vi "pop_nil.vi"(8 "error in (no error)":errorcluster, 11 "Lua in":refnum<class "Lua.lvclass">) -> (0 "error out":errorcluster, 2 "value (ignored)":bool, 3 "Lua out":refnum<class "Lua.lvclass">)   [LabVIEW 2020, in "Lua for LabVIEW.lvlib" / "Lua.lvclass"]
doc: "Pop any value from the stack without returning the result."
uses:
  Lua.lvclass
  Lua.lvclass/Lua.ctl
  lib/lua.dll/lua.dll.lvlib
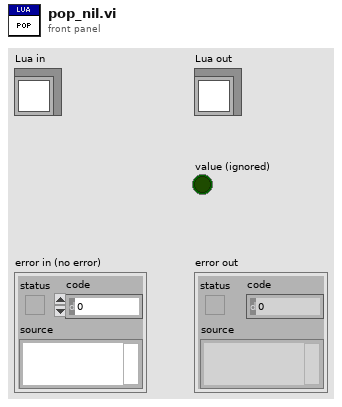
[diagram p1: front panel]
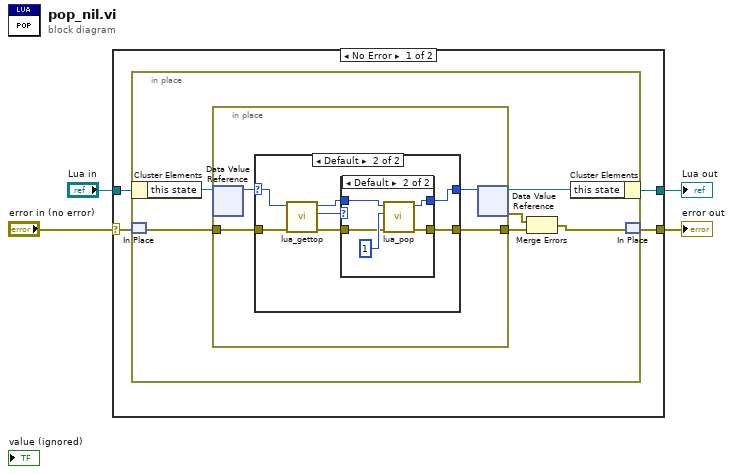
[diagram p0: block diagram]
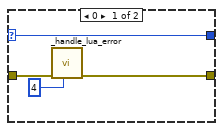
[diagram p2: hidden frame]
diagram:
  n1 = case shown="No Error" "error in (no error)" {
    selector: "error in (no error)" -> [w5 w38]
    tunnel: [w6 w38] -> w3
    tunnel: [w7 w37] -> w1
    tunnel: "Lua in" -> [w8 w37]
    frame No Error {
      n2 = in-place {
        n3 = in-place-cluster #1(w8) -> ("this state"=w13:refnum<data-value>)
        n4 = in-place-match #2(w5) -> (w14:errorcluster)
        n5 = in-place {
          in-place-border: w14 -> [w18]
          in-place-border: [w15] -> w9
          n6 = in-place-dvr #3(w13) -> (w17:u64)  [unwired: 1 out]
          n7 = case shown="Default" w17 {
            selector: w17 -> [w22 w26]
            tunnel: [w22 w28] -> w16
            tunnel: w18 -> [w19 w27]
            tunnel: [w20 w29] -> w15
            frame 0 {
              n8 = call "_handle_lua_error.vi"("lua status"=4 ("lua_load errcode"), "error in (no error)"=w19) -> ("error out"=w20:errorcluster)  [unwired: 9 in]
            }
            frame Default {
              n9 = call "lua_gettop.vi"("error in (no error)"=w27, "lua_state_p"=w26) -> ("error out"=w25:errorcluster, "index"=w24:i32, "lua_state_p out"=w23:u64)  [unwired: 7 in]
              n10 = case shown="Default" w24 {
                tunnel: [w31 w36] -> w29
                tunnel: [w30 w35] -> w28
                tunnel: w25 -> [w31 w33]
                tunnel: w23 -> [w30 w32]
                frame 0 {
                }
                frame Default {
                  n11 = call "lua_pop.vi"("error in (no error)"=w33, "n"=1 ("index"), "lua_state_p"=w32) -> ("error out"=w36:errorcluster, "lua_state_p out"=w35:u64)  [unwired: 7 in]
                }
              }
            }
          }
          n12 = in-place-dvr #3(w16) -> (w12:refnum<data-value>, w11:errorcluster)
        }
        n13 = Merge Errors(w11, w9) -> (w10:errorcluster)
        n14 = in-place-cluster #1("this state"=w12) -> (w7:refnum<class "Lua.lvclass">)
        n15 = in-place-match #2(w10) -> (w6:errorcluster)
      }
    }
    frame Error {
    }
  }
  "error out" <- w3
  "Lua out" <- w1
